vi "niScope Multi Read WDT.vi"(5 "timestamp Type":T1=1 caption="timestamp type" items=["relative", "absolute"], 7 "timeout":dbl=5.0 format="%.2f", 8 "error in":errorcluster, 9 "numSamples":i32=-1, 10 "channels":string="0", 11 "instrument handle":refnum<k15>) -> (0 "error out":errorcluster, 1 "wfm":waveform(dbl)[](array[waveform]), 2 "wfm info":T2(array[cluster]) {"reserved2" format="%.2f"; "reserved1" format="%.2f"; "offset" format="%^.3e"; "gain" format="%^.3e"; "xIncrement" format="%^.3e"; "relativeInitialX" format="%^.3e"; "absoluteInitialX" format="%^.3e"}, 3 "instrument handle out":refnum<k15>)   [LabVIEW 2011]
doc: "Initiates an acquisition and returns a one-dimensional array of LabVIEW waveform data types that includes timing information. This VI is only supported in LabVIEW 7.0 or later."
uses:
  <instrlib>/niScope/Controls/niScope timestamp type.ctl
  niScope_32.dll
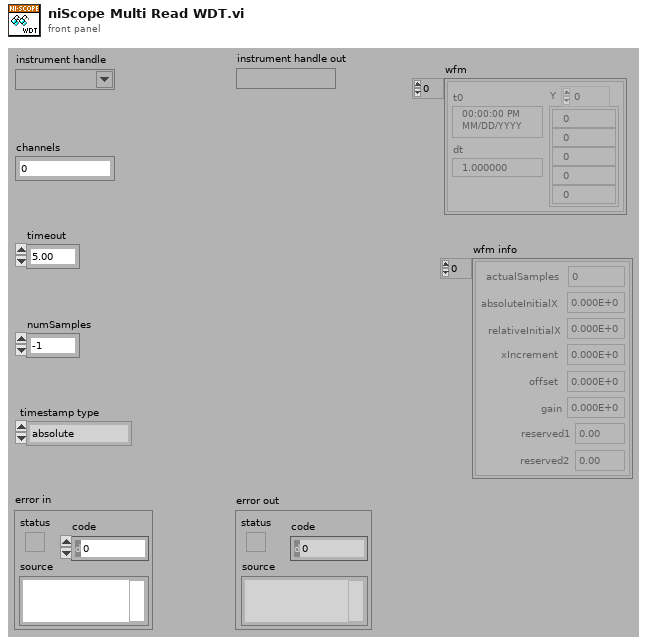
[diagram p1: front panel]
types:
  T1 = typedef "niScope timestamp type.ctl" = i32
  T2 = cluster{"actualSamples":i32, "absoluteInitialX":dbl, "relativeInitialX":dbl, "xIncrement":dbl, "offset":dbl, "gain":dbl, "reserved1":dbl, "reserved2":dbl}[]
  T3 = cluster{"actualSamples":i32, "absoluteInitialX":dbl, "relativeInitialX":dbl, "xIncrement":dbl, "offset":dbl, "gain":dbl, "reserved1":dbl, "reserved2":dbl}
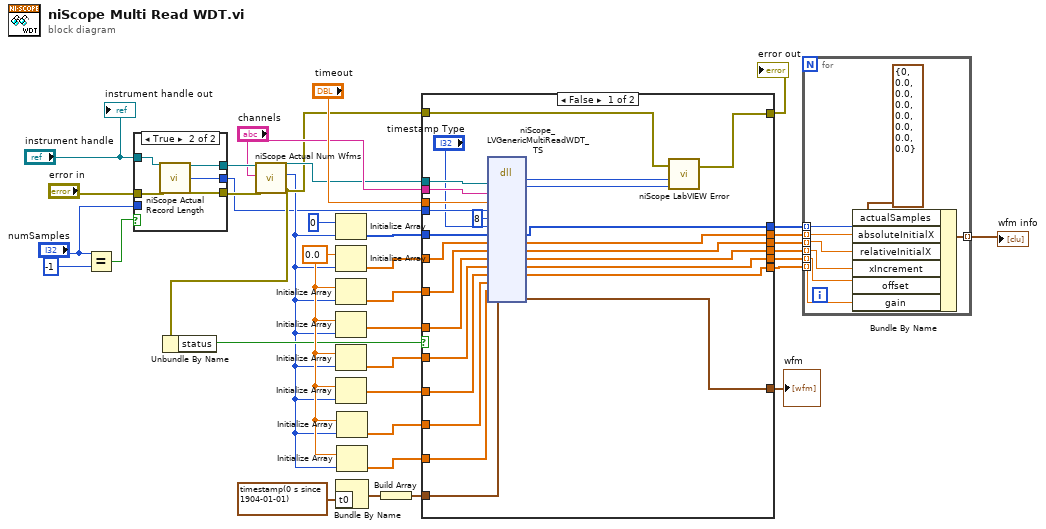
[diagram p0: block diagram]
diagram:
  w30 = 0.0 ("Element Data")
  n1 = Equal?(x="numSamples", y=-1) -> (x = y?=w35:bool)
  n2 = case shown="True" w35 {
    tunnel: [w37 w44] -> w32
    tunnel: [w38 w43] -> w33
    tunnel: "numSamples" -> [w39 _]
    tunnel: [w39 w42] -> w7
    tunnel: "instrument handle" -> [w38 w41]
    tunnel: "error in" -> [w37 w40]
    frame False {
    }
    frame True {
      n3 = call <instrlib>:"niScope Actual Record Length.vi"("instrument handle"=w41, "error in"=w40) -> ("instrument handle out"=w43:refnum<k15>, "actual record length"=w42:i32, "error out"=w44:errorcluster)  [unwired: 11 in]
    }
  }
  n4 = call <instrlib>:"niScope Actual Num Wfms.vi"("error in"=w32, "channels"="channels", "instrument handle"=w33) -> ("error out"=w9:errorcluster, "actual num wfms"=w8:i32, "instrument handle out"=w19:refnum<k15>)  [unwired: 6 in]
  n5 = Unbundle By Name(w9) -> ("status"=w18:bool)
  n6 = Initialize Array(0 ("Element Data"), w8) -> (w22:i32[])
  n7 = Initialize Array(w30, w8) -> (w23:dbl[])
  n8 = Initialize Array(w30, w8) -> (w24:dbl[])
  n9 = Initialize Array(w30, w8) -> (w25:dbl[])
  n10 = Initialize Array(w30, w8) -> (w26:dbl[])
  n11 = Initialize Array(w30, w8) -> (w27:dbl[])
  n12 = Bundle By Name("t0"=timestamp(0 s since 1904-01-01)) -> (w2:waveform(dbl))  [unwired: 1 in]
  n13 = Initialize Array(w30, w8) -> (w28:dbl[])
  n14 = Initialize Array(w30, w8) -> (w29:dbl[])
  n15 = Build Array(w2) -> (w1:waveform(dbl)[])
  n16 = case shown="False" w18 {
    tunnel: w29 -> [w60 _]
    tunnel: w28 -> [w59 _]
    tunnel: w27 -> [w58 w72]
    tunnel: w26 -> [w57 w73]
    tunnel: w25 -> [w56 w74]
    tunnel: w24 -> [w55 w75]
    tunnel: w23 -> [w54 w76]
    tunnel: w22 -> [w53 w77]
    tunnel: w7 -> [w69 _]
    tunnel: "timeout" -> [w68 _]
    tunnel: "channels" -> [w67 _]
    tunnel: w19 -> [w66 _]
    tunnel: [w52 w72] -> w17
    tunnel: [w51 w73] -> w16
    tunnel: [w50 w74] -> w15
    tunnel: [w49 w75] -> w14
    tunnel: [w48 w76] -> w12
    tunnel: [w47 w77] -> w13
    tunnel: [w63 w78] -> w10
    tunnel: w9 -> [w62 w78]
    tunnel: [w61 w71] -> w4
    tunnel: w1 -> [w45 w71]
    frame False {
      n17 = dll-call lib="niScope_*.*" fn="niScope_LVGenericMultiReadWDT_TS"("instrument handle"=w66, "channelList"=w67, "timeout"=w68, "numSamples"=w69, "dataType"=8, "timestampType"="timestamp Type", "actualSamples"=w53, "absoluteInitialX"=w54, "relativeInitialX"=w55, "xIncrement"=w56, "offset"=w57, "gain"=w58, "reserved1"=w59, "reserved2"=w60, "wfm"=w45) -> ("status"=w65:i32, "instrument handle"=w64:u32, "actualSamples"=w47:i32[], "absoluteInitialX"=w48:dbl[], "relativeInitialX"=w49:dbl[], "xIncrement"=w50:dbl[], "offset"=w51:dbl[], "gain"=w52:dbl[], "wfm"=w61:waveform(dbl)[])  [unwired: 10 in, 2 out]
      n18 = call <instrlib>:"niScope LabVIEW Error.vi"("instrument handle"=w64, "niScope error code (0)"=w65, "error in (no error)"=w62) -> ("error out"=w63:errorcluster)  [unwired: 2 in]
    }
    frame True {
    }
  }
  "error out" <- w10
  "wfm" <- w4
  n19 = for {
    tunnel: w14 -> [w80] mode=indexing
    tunnel: w15 -> [w81] mode=indexing
    tunnel: w16 -> [w84] mode=indexing
    tunnel: w17 -> [w83] mode=indexing
    tunnel: w13 -> [w79] mode=indexing
    tunnel: w12 -> [w85] mode=indexing
    tunnel: [w82] -> w11 mode=indexing
    n20 = Bundle By Name(cluster=T3 {"actualSamples"=0, "absoluteInitialX"=0.0, "relativeInitialX"=0.0, "xIncrement"=0.0, "offset"=0.0, "gain"=0.0, "reserved1"=0.0, "reserved2"=0.0}, "actualSamples"=w79, "absoluteInitialX"=w85, "relativeInitialX"=w80, "xIncrement"=w81, "offset"=w84, "gain"=w83) -> (w82:T3)
  }
  "wfm info" <- w11
  "instrument handle out" <- "instrument handle"
